vi "user32_ReleaseCapture.vi"(8 "error in (no error)":errorcluster) -> (0 "error out":errorcluster, 3 "Return Value":i32)   [LabVIEW 2020]
uses:
  user32.dll
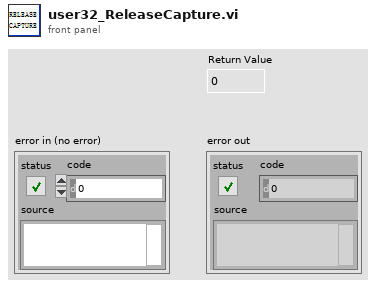
[diagram p1: front panel]
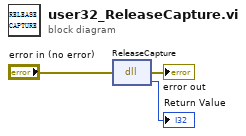
[diagram p0: block diagram]
diagram:
  n1 = dll-call lib="user32.dll" fn="ReleaseCapture"(error in="error in (no error)") -> (error out=→"error out":errorcluster, "返回值"=→"Return Value":i32)  [unwired: 2 in, 1 out]
